vi "SeqMgr.Compare Param Values.vi"(8 "error in":errorcluster, 11 "Var,Comp,Var":string[](array[string])) -> (0 "error out":errorcluster, 3 "Boolean":bool)   [LabVIEW 2024, in "EQMF.lvlib" / "SeqMgr.lvlib"]
uses:
  SeqMgr.lvlib
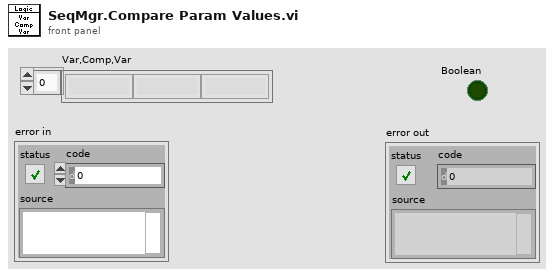
[diagram p1: front panel]
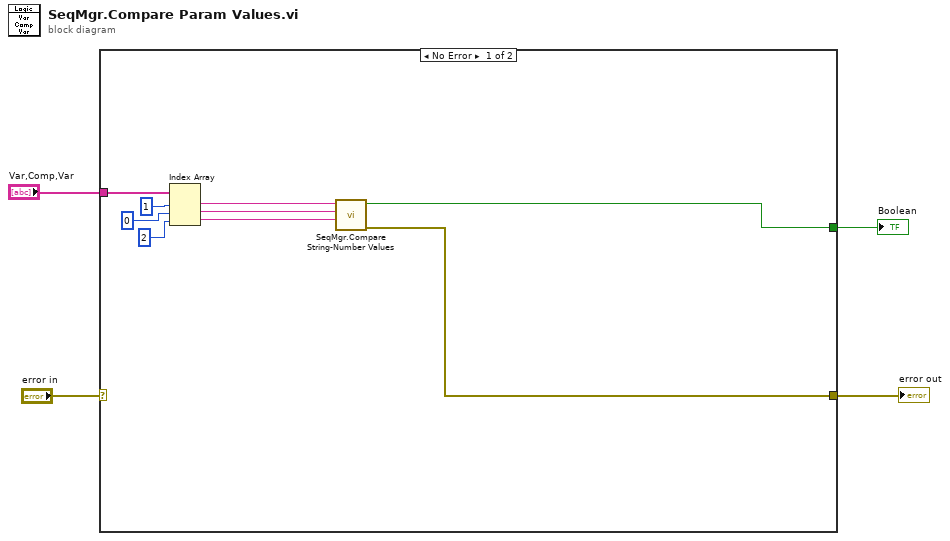
[diagram p0: block diagram]
diagram:
  n1 = case shown="No Error" "error in" {
    selector: "error in" -> [_ w14]
    tunnel: "Var,Comp,Var" -> [w13 _]
    tunnel: [w5 w14] -> w2
    tunnel: [w6 _] -> w1
    frame No Error {
      n2 = Index Array(array=w13, index #1=1 ("index"), index #2=0 ("index"), index #3=2 ("index")) -> (element #1=w9:string, element #2=w8:string, element #3=w7:string)
      n3 = call "SeqMgr.Compare String-Number Values.vi"("Input 2"=w7, "Input 1"=w8, "Comparison"=w9) -> ("error"=w5:errorcluster, "T/F"=w6:bool)  [unwired: 6 in, 1 out]
    }
    frame Error {
    }
  }
  "Boolean" <- w1
  "error out" <- w2
